vi "Format Evaluation into File Format.vi"(8 "error in (no error)":errorcluster, 10 "Evaluation":T1 {"Low Limit" format="%#_13g"; "SI Scaling" items=["femto"=-15, "pico"=-12, "nano"=-9, "micro"=-6, "milli"=-3, "percent"=-2, ""=0, "kilo"=3, "mega"=6, "giga"=9, "tera"=12]}, 11 "Test Modes":string[](array[string])) -> (0 "error out":errorcluster, 2 "Row Data Out":string[](array[string]))   [LabVIEW 2018, in "Test Number and Bin Generator.lvlib" / "Test Number and Bin Generator.lvclass"]
uses:
  Test Number and Bin Generator.lvclass
  Plugins/TestStand API Tools (TSAT).lvlibp/Evaluation Actions/Includes/Controls/TSAT Evaluation.ctl
  Plugins/TestStand API Tools (TSAT).lvlibp/Evaluation Actions/Includes/Controls/TSAT Eval SI Unit Scaling.ctl
  Plugins/TestStand API Tools (TSAT).lvlibp/Evaluation Actions/Includes/Controls/TSAT Evaluation Type.ctl
  Plugins/TestStand API Tools (TSAT).lvlibp/Evaluation Actions/TSAT Evaluation Actions.lvlib
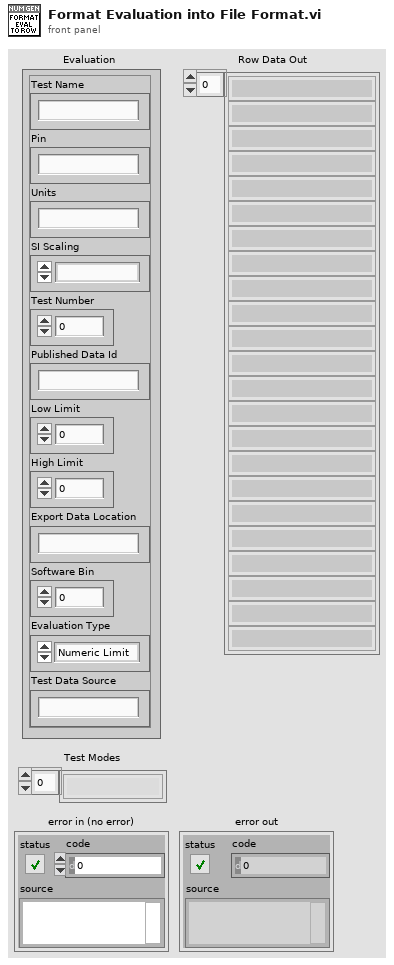
[diagram p1: front panel]
types:
  T1 = typedef "TestStand API Tools (TSAT).lvlibp/TSAT Evaluation Actions.lvlib/TSAT Evaluation.ctl" = cluster{"Test Name":string, "Pin":string, "Units":string, "SI Scaling":T2, "Test Number":i32, "Published Data Id":string, "Low Limit":dbl, "High Limit":dbl, "Export Data Location":string, "Software Bin":i64, "Evaluation Type":T3, "Test Data Source":string}
  T2 = typedef "TestStand API Tools (TSAT).lvlibp/TSAT Evaluation Actions.lvlib/TSAT Eval SI Unit Scaling.ctl" = i16
  T3 = typedef "TestStand API Tools (TSAT).lvlibp/TSAT Evaluation Actions.lvlib/TSAT Evaluation Type.ctl" = enum16{"Numeric Limit", "Pass/Fail", "None"}
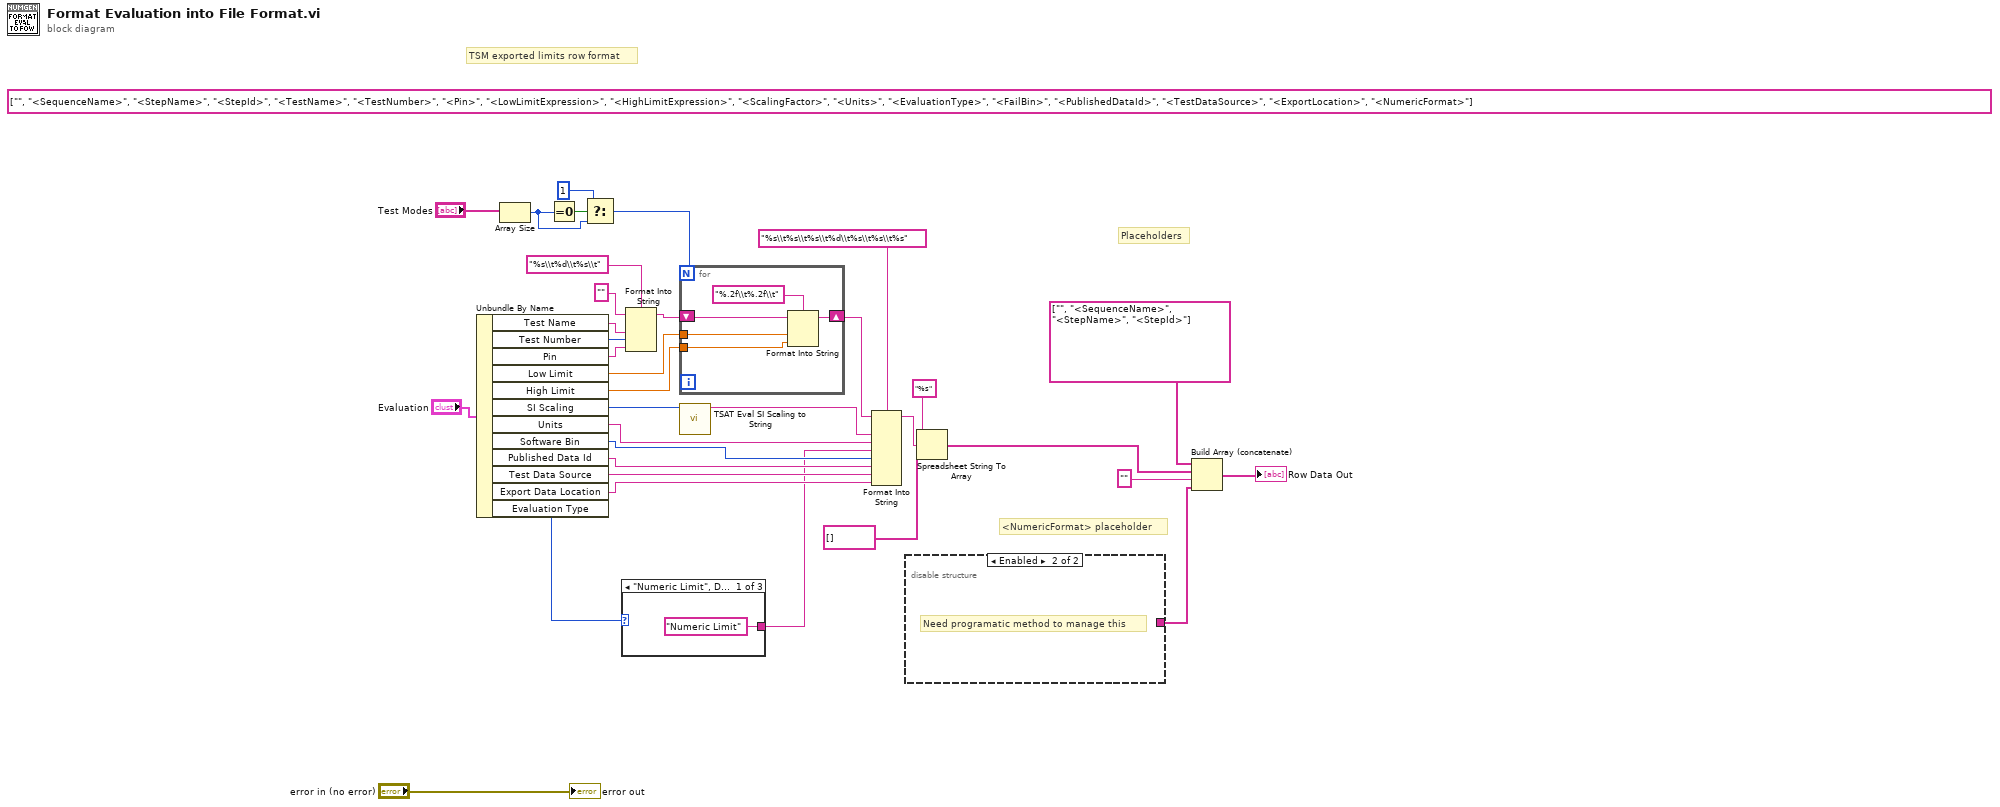
[diagram p0: block diagram]
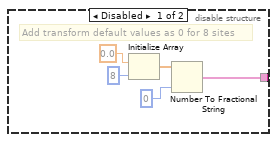
[diagram p2: hidden frame]
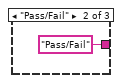
[diagram p3: hidden frame]
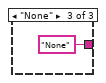
[diagram p4: hidden frame]
diagram:
  (unwired) string[] ["", "<SequenceName>", "<StepName>", "<StepId>", "<TestName>", "<TestNumber>", "<Pin>", "<LowLimitExpression>", "<HighLimitExpression>", "<ScalingFactor>", "<Units>", "<EvaluationType>", "<FailBin>", "<PublishedDataId>", "<TestDataSource>", "<ExportLocation>", "<NumericFormat>"] ("Array")
  # "Placeholders"
  # "<NumericFormat> placeholder"
  # "TSM exported limits row format"
  n1 = Unbundle By Name("Evaluation") -> ("Test Name"=w33:string, "Test Number"=w32:i32, "Pin"=w31:string, "Low Limit"=w30:dbl, "High Limit"=w29:dbl, "SI Scaling"=w25:T2, "Units"=w22:string, "Software Bin"=w14:i64, "Published Data Id"=w21:string, "Test Data Source"=w20:string, "Export Data Location"=w11:string, "Evaluation Type"=w2:T3)
  n2 = Array Size(array="Test Modes") -> (size(s)=w8:i32)
  n3 = Equal To 0?(x=w8) -> (x = 0?=w9:bool)
  n4 = Select(t=1, s=w9, f=w8) -> (s? t:f=w6:i32)
  n5 = case shown="\"Numeric Limit\", Default" w2 {
    tunnel: ["Numeric Limit" ("input 4") "Pass/Fail" ("input 4") "None" ("input 4")] -> w1
    frame "Numeric Limit", Default {
    }
    frame "Pass/Fail" {
    }
    frame "None" {
    }
  }
  n6 = Format Into String(format string="%s\\t%d\\t%s\\t", initial string="", w33, w32, w31) -> (resulting string=w27:string)  [unwired: 1 in, 1 out]
  n7 = for {
    N: w6 -> [_]
    tunnel: w30 -> [w42]
    tunnel: w29 -> [w41]
    shift-right: [w39] -> w26
    shift-left: w27 -> [w40]
    n8 = Format Into String(format string="%.2f\\t%.2f\\t", initial string=w40, w42, w41) -> (resulting string=w39:string)  [unwired: 1 in, 1 out]
  }
  n9 = call "TSAT Eval SI Scaling to String.vi"("SI Scaling"=w25) -> ("String"=w23:string)  [unwired: 10 in]
  n10 = Format Into String(format string="%s\\t%s\\t%s\\t%d\\t%s\\t%s\\t%s", initial string=w26, w23, w22, w1, w14, w21, w20, w11) -> (resulting string=w18:string)  [unwired: 1 in, 1 out]
  n11 = disable-structure shown="Enabled" {
    disable-tunnel: [w43 _] -> w5
    frame Disabled {
      # "Add transform default values as 0 for 8 sites"
      n12 = Initialize Array(0.0 ("dimension size"), 8 ("dimension size")) -> (w45:dbl[])
      n13 = Number To Fractional String(number=w45, precision (6)=i16 0) -> (F-format string=w43:string[])  [unwired: 2 in]
    }
    frame Enabled {
      # "Need programatic method to manage this"
    }
  }
  n14 = Spreadsheet String To Array(format string="%s", spreadsheet string=w18, array type (2D Dbl)=string[] []) -> (array=w13:string[])  [unwired: 1 in]
  n15 = Build Array (concatenate)(string[] ["", "<SequenceName>", "<StepName>", "<StepId>"] ("array"), w13, "", w5) -> (→"Row Data Out":string[])
  "error out" <- "error in (no error)"
